vi "Get Windows Process Memory Usage.vi"() -> (3 "Memory Used By This Process (KB)":dbl)   [LabVIEW 2021]
panel:
  out "x/y":dbl format="%.3f"
  in  "stop":bool
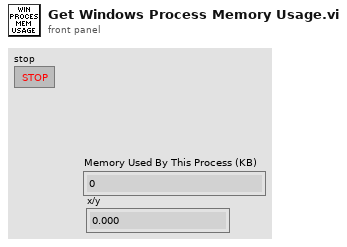
[diagram p1: front panel]
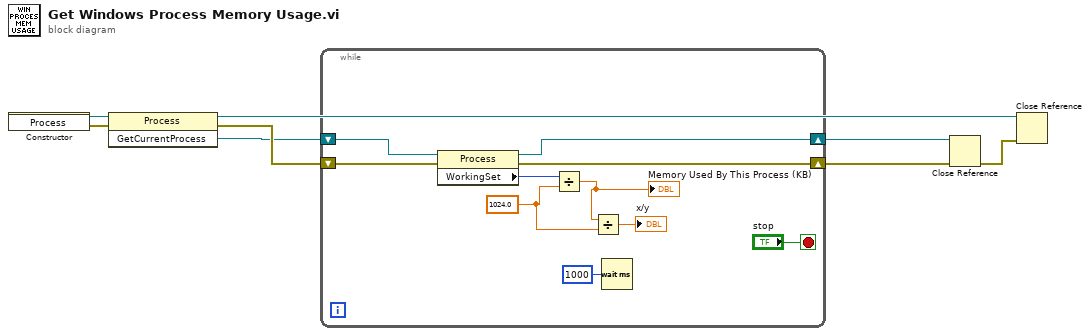
[diagram p0: block diagram]
diagram:
  n1 = constructor class="Process"() -> (reference out=w8:refnum<k24>, error out=w1:errorcluster)  [unwired: 3 in, 1 out]
  n2 = invoke class="Process" method="GetCurrentProcess"(reference=w8, error in=w1) -> (reference out=w6:refnum<k24>, error out=w7:errorcluster, "GetCurrentProcess"=w2:refnum<k24>)  [unwired: 1 in]
  n3 = while {
    shift-right: [w16] -> w3
    shift-left: w7 -> [w18]
    shift-right: [w17] -> w4
    shift-left: w2 -> [w14]
    stop <- "stop" stop-if-true
    w10 = 1024.0 ("y")
    n4 = property class="Process"(reference=w14, error in=w18) -> (reference out=w17:refnum<k24>, error out=w16:errorcluster, "WorkingSet"=w15:i32)
    n5 = Divide(x=w15, y=w10) -> (x/y=w11:dbl)
    "Memory Used By This Process (KB)" <- w11
    n6 = Divide(x=w11, y=w10) -> (x/y=→"x/y":dbl)
    n7 = Wait (ms)(milliseconds to wait=u32 1000) -> ()  [unwired: 1 out]
  }
  n8 = Close Reference(reference=w4, error in (no error)=w3) -> (error out=w5:errorcluster)
  n9 = Close Reference(reference=w6, error in (no error)=w5) -> ()  [unwired: 1 out]
